vi "RD Digital IO Output Enable Set.vi"(8 "error in (no error)":errorcluster caption="错误输入（无错误）", 10 "outputs":u32, 11 "handle":u32) -> (0 "error out":errorcluster caption="错误输出", 2 "function return":i32, 3 "handle out":u32)   [LabVIEW 2018, in "InstrumentsPlayground.lvlib"]
doc: "CLIFFAPI int CliffDigitalIOOutputEnableSet(FT_HANDLE handle,uint outputs);"
uses:
  InstrumentsPlayground.lvlib
  InstrumentsPlayground.dll
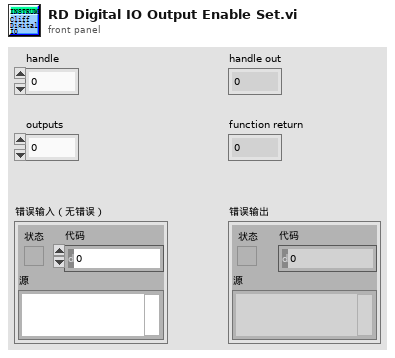
[diagram p1: front panel]
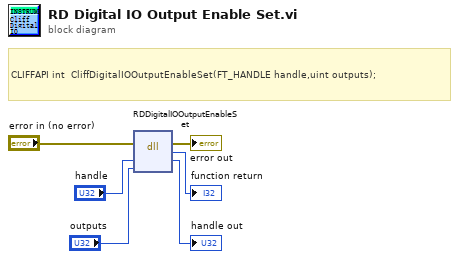
[diagram p0: block diagram]
diagram:
  # "CLIFFAPI int  CliffDigitalIOOutputEnableSet(FT_HANDLE handle,uint outputs);"
  n1 = dll-call lib="E:/Work/YZCourse_Xtext/Cliff/API/IPLabView lib/InstrumentsPlayground.*" fn="RDDigitalIOOutputEnableSet"(error in="error in (no error)", "handle"="handle", "outputs"="outputs") -> (error out=→"error out":errorcluster, "返回类型"=→"function return":i32, "handle"=→"handle out":u32)  [unwired: 3 in, 1 out]
